vi "setILCMap.vi"(10 "ILCMap":T1[][](array[typedef]), 11 "ILCCommunications in":refnum<class "ILCCommunications.lvclass">) -> (3 "ILCCommunications out":refnum<class "ILCCommunications.lvclass">)   [LabVIEW 2016, in "ILCCommunications.lvclass"]
uses:
  ILCCommunications.lvclass
  Types/ILCMap.ctl
  Types/ILCTypes.ctl
  ILCCommunications.lvclass/ILCCommunications.ctl
  Types/M1M3SupportTypes.lvlib
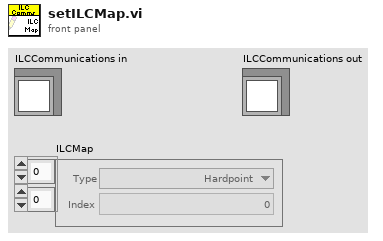
[diagram p1: front panel]
types:
  T1 = typedef "M1M3SupportTypes.lvlib/ILCMap.ctl" = cluster{"Index":i32, "Type":T2}
  T2 = typedef "M1M3SupportTypes.lvlib/ILCTypes.ctl" = enum16{"Hardpoint", "Force"}
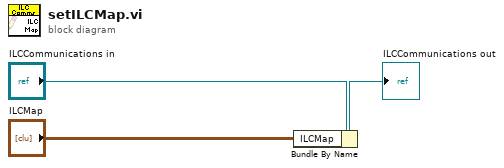
[diagram p0: block diagram]
diagram:
  n1 = Bundle By Name(cluster="ILCCommunications in", "ILCMap"="ILCMap") -> (→"ILCCommunications out":refnum<class "ILCCommunications.lvclass">)
